vi "CC Script Parse Acquire Images.vi"(8 "error in (no error)":errorcluster, 9 "To Script?":bool, 10 "Acquire Parameters in":T1, 11 "DefineObject Parameters":string="Exposure=\"Exposure Test\", Object=\"This is my object\", Dithering=\"Some sort of dither\"") -> (0 "error out":errorcluster, 2 "Script out":string="ObjectName \"RA\":\"123.456\",\"DEC\":\"4546.54\"", 3 "Acquire Parameters":T1)   [LabVIEW 2024]
uses:
  typedefs/CC cluster Acquire Parameters.ctl
  <vilib>/Utility/error.llb/Trim Whitespace One-Sided.vi
  <vilib>/regexp/Match Regular Expression.xnode
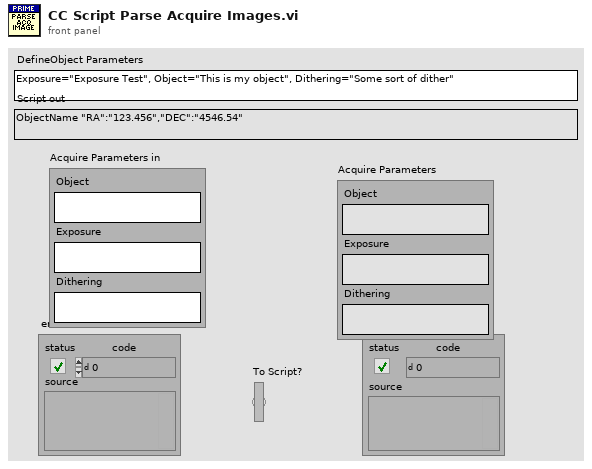
[diagram p1: front panel]
types:
  T1 = typedef "CC cluster Acquire Parameters.ctl" = cluster{"Object":string, "Exposure":string, "Dithering":string}
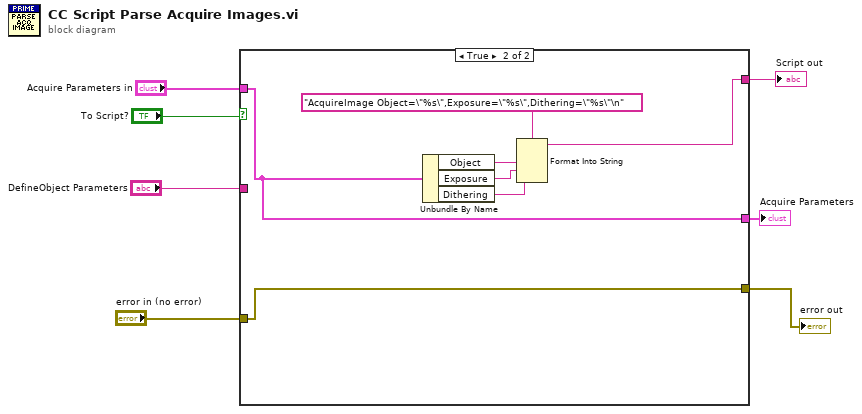
[diagram p0: block diagram]
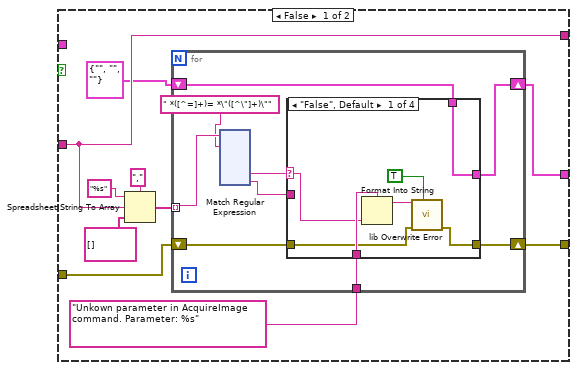
[diagram p2: hidden frame]
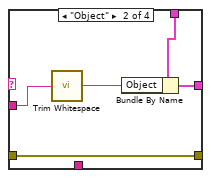
[diagram p3: hidden frame]
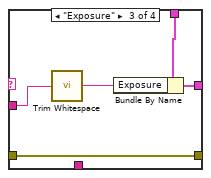
[diagram p4: hidden frame]
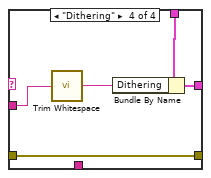
[diagram p5: hidden frame]
diagram:
  n1 = case shown="True" "To Script?" {
    tunnel: "DefineObject Parameters" -> [w14 _]
    tunnel: [w11 w170] -> w6
    tunnel: "Acquire Parameters in" -> [_ w170]
    tunnel: [w14 w171] -> w3
    tunnel: "error in (no error)" -> [w10 w169]
    tunnel: [w8 w169] -> w1
    frame False {
      n2 = Spreadsheet String To Array(delimiter (Tab)=",", format string="%s", spreadsheet string=w14, array type (2D Dbl)=string[] []) -> (array=w12:string[])
      n3 = for {
        shift-right: [w22] -> w11
        shift-left: T1 {"Object"="", "Exposure"="", "Dithering"=""} ("Acquire Parameters") -> [w26]
        tunnel: w12 -> [w25] mode=indexing
        shift-right: [w18] -> w8
        shift-left: w10 -> [w19]
        tunnel: "Unkown parameter in AcquireImage command. Parameter: %s" ("format string") -> [w20]
        n4 = xnode "Match Regular Expression"("input string"=w25, "regular expression"=" *([^=]+)= *\"([^\"]+)\"" ("format string")) -> ("submatch 1"=w24:string, "submatch 2"=w23:string)  [unwired: 4 in, 5 out]
        n5 = case shown="\"False\", Default" w24 {
          selector: w24 -> [w31 _ _ _]
          tunnel: [w33 w38 w43 w48] -> w22
          tunnel: w26 -> [w33 w36 w41 w46]
          tunnel: w23 -> [_ w35 w40 w45]
          tunnel: w20 -> [w32 _ _ _]
          tunnel: w19 -> [w29 w34 w39 w44]
          tunnel: [w27 w34 w39 w44] -> w18
          frame "False", Default {
            n6 = Format Into String(format string=w32, w31) -> (resulting string=w30:string)  [unwired: 2 in, 1 out]
            n7 = call "lib Overwrite Error.vi"("Force Error?"=TRUE, "error in (no error)"=w29, "Error Message"=w30) -> ("error out"=w27:errorcluster)  [unwired: 8 in]
          }
          frame "Object" {
            n8 = call <vilib>:"Trim Whitespace.vi"("string"=w35) -> ("trimmed string"=w37:string)  [unwired: 1 in]
            n9 = Bundle By Name(cluster=w36, "Object"=w37) -> (w38:T1)
          }
          frame "Exposure" {
            n10 = call <vilib>:"Trim Whitespace.vi"("string"=w40) -> ("trimmed string"=w42:string)  [unwired: 1 in]
            n11 = Bundle By Name(cluster=w41, "Exposure"=w42) -> (w43:T1)
          }
          frame "Dithering" {
            n12 = call <vilib>:"Trim Whitespace.vi"("string"=w45) -> ("trimmed string"=w47:string)  [unwired: 1 in]
            n13 = Bundle By Name(cluster=w46, "Dithering"=w47) -> (w48:T1)
          }
        }
      }
    }
    frame True {
      n14 = Unbundle By Name(w170) -> ("Object"=w174:string, "Exposure"=w173:string, "Dithering"=w172:string)
      n15 = Format Into String(format string="AcquireImage Object=\"%s\",Exposure=\"%s\",Dithering=\"%s\"\n", w174, w173, w172) -> (resulting string=w171:string)  [unwired: 2 in, 1 out]
    }
  }
  "error out" <- w1
  "Acquire Parameters" <- w6
  "Script out" <- w3
